vi "Units Quantum Example.vi"(8 "error in (no error)":errorcluster) -> (0 "error out":errorcluster)   [LabVIEW 2020]
uses:
  Type Definitions/UNIST Fluid Rate.ctl
panel:
  in  "milliseconds to wait":u32=5000
  in  "Fluid Rate (CC/MIN)":T1="080"
  in  "Clear Alarm":bool
  in  "VISA resource name":refnum<visa-resource-name>
  # "PORT 4: = Quantum Oil Injection Machine"
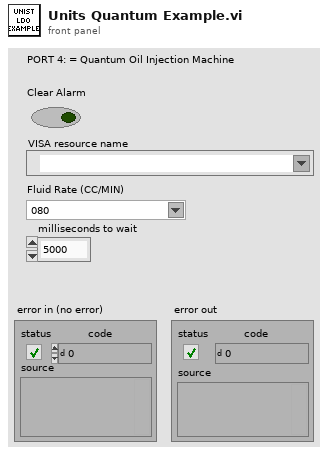
[diagram p1: front panel]
types:
  T1 = typedef "UNIST Fluid Rate.ctl" = string
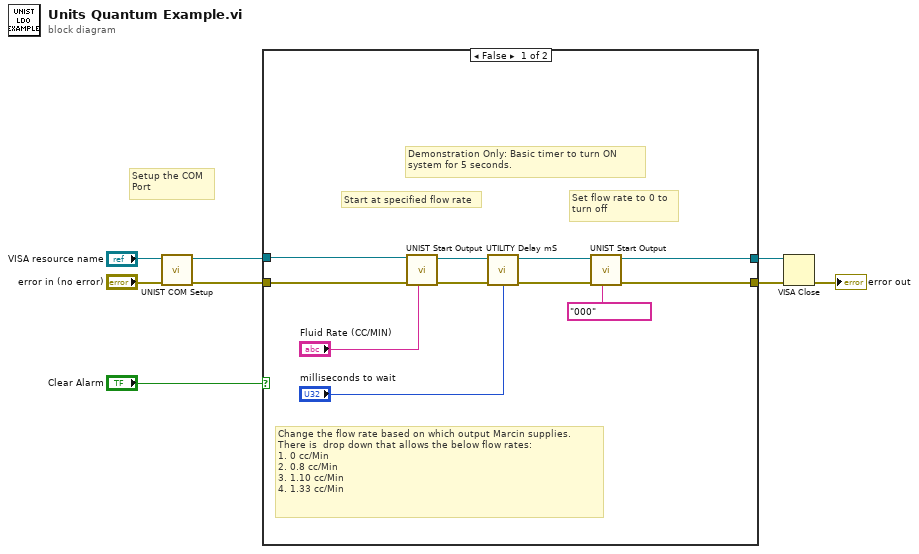
[diagram p0: block diagram]
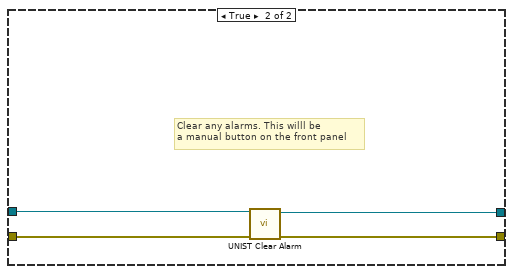
[diagram p2: hidden frame]
diagram:
  # "Setup the COM\nPort"
  n1 = call "UNIST COM Setup.vi"("error in (no error)"="error in (no error)", "VISA Refnum in"="VISA resource name") -> ("error out"=w2:errorcluster, "VISA Refnum out"=w3:refnum<visa-resource-name>)  [unwired: 8 in]
  n2 = case shown="False" "Clear Alarm" {
    tunnel: [w10 w20] -> w5
    tunnel: [w9 w19] -> w4
    tunnel: w3 -> [w18 w21]
    tunnel: w2 -> [w17 w22]
    frame False {
      # "Change the flow rate based on which output Marcin supplies.\nThere is  drop down that allows the below flow rates:\n1. 0 cc/Min\n2. 0.8 cc/Min\n3. 1.10 cc/Min\n4. 1.33 cc/Min"
      # "Demonstration Only: Basic timer to turn ON\nsystem for 5 seconds."
      # "Set flow rate to 0 to \nturn off"
      # "Start at specified flow rate"
      n3 = call "UNIST Start Output.vi"("Fluid Rate (CC/MIN)"="Fluid Rate (CC/MIN)", "error in (no error)"=w17, "VISA Refnum in"=w18) -> ("error out"=w15:errorcluster, "VISA Refnum out"=w14:refnum<visa-resource-name>)  [unwired: 7 in]
      n4 = call "UTILITY Delay mS.vi"("Error In"=w15, "milliseconds to wait"="milliseconds to wait") -> ("Error Out"=w13:errorcluster)  [unwired: 13 in]
      n5 = call "UNIST Start Output.vi"("Fluid Rate (CC/MIN)"=T1 "000", "error in (no error)"=w13, "VISA Refnum in"=w14) -> ("error out"=w9:errorcluster, "VISA Refnum out"=w10:refnum<visa-resource-name>)  [unwired: 7 in]
    }
    frame True {
      # "Clear any alarms. This willl be\na manual button on the front panel"
      n6 = call "UNIST Clear Alarm.vi"("error in (no error)"=w22, "VISA Refnum in"=w21) -> ("error out"=w19:errorcluster, "VISA Refnum out"=w20:refnum<visa-resource-name>)  [unwired: 8 in]
    }
  }
  n7 = VISA Close(VISA resource name=w5, error in (no error)=w4) -> (error out=→"error out":errorcluster)
